vi "GUIReferences.vi"(7 "Action":T1, 8 "error in (no error)":errorcluster, 10 "String":string, 11 "VI Refnum":refnum<vi>) -> (0 "error out":errorcluster, 3 "VI Refnum":refnum<vi>)   [LabVIEW 2017, in "MainGUI.lvlib"]
uses:
  MainGUI.lvlib
  GUIReferences.Action.ctl
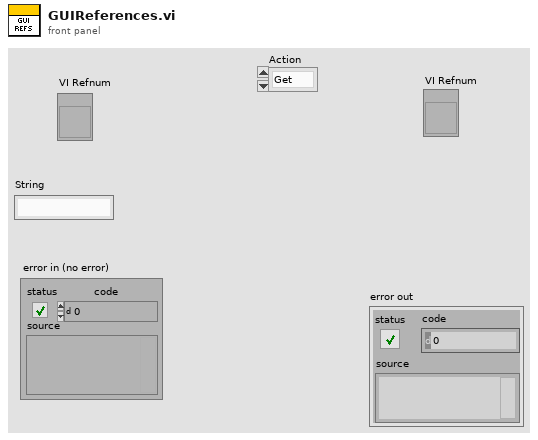
[diagram p1: front panel]
types:
  T1 = typedef "MainGUI.lvlib/GUIReferences.Action.ctl" = enum16{"Get", "Register", "Unregister"}
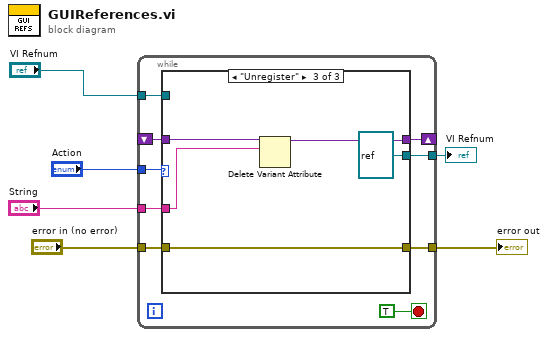
[diagram p0: block diagram]
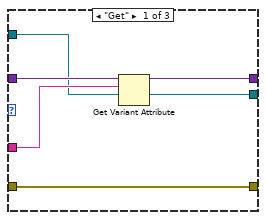
[diagram p2: hidden frame]
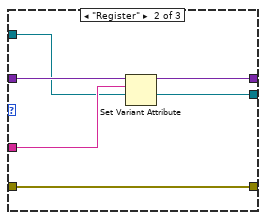
[diagram p3: hidden frame]
diagram:
  n1 = while {
    tunnel: "VI Refnum" -> [w9]
    tunnel: "Action" -> [w14]
    shift-right: [w13] -> _
    shift-left: _ -> [w8]
    tunnel: "error in (no error)" -> [w12]
    tunnel: [w11] -> w3
    tunnel: "String" -> [w10]
    tunnel: [w7] -> w1
    stop <- TRUE stop-if-true
    n2 = case shown="\"Unregister\"" w14 {
      tunnel: [w18 w26 w30] -> w13
      tunnel: w12 -> [w16 w25 w28]
      tunnel: [w16 w25 w28] -> w11
      tunnel: w10 -> [w20 w24 w29]
      tunnel: w9 -> [w19 w22 _]
      tunnel: w8 -> [w21 w23 w31]
      tunnel: [w17 w22 refnum<vi> refnum ("VI Refnum")] -> w7
      frame "Get" {
        n3 = Get Variant Attribute(Variant=w21, name=w20, default value (empty Variant)=w19) -> (duplicate Variant=w18:variant, value=w17:refnum<vi>)  [unwired: 1 in, 2 out]
      }
      frame "Register" {
        n4 = Set Variant Attribute(Variant=w23, name=w24, value=w22) -> (Variant out=w26:variant)  [unwired: 1 in, 2 out]
      }
      frame "Unregister" {
        n5 = Delete Variant Attribute(6:w29, 7:w31) -> (3:w30:variant)  [unwired: 1 in, 2 out]
      }
    }
  }
  "error out" <- w3
  "VI Refnum" <- w1
